vi "trmm - Triangle Matrix-Matrix Product.vi"   [LabVIEW 2020, in "NI_AALBLAS.lvlib"]
doc: "Calculates the product of a triangular matrix and another matrix."
uses:
  NI_AALBLAS.lvlib
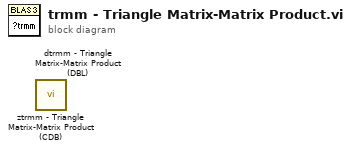
[diagram p0: block diagram]
diagram:
  n1 = call "ztrmm - Triangle Matrix-Matrix Product (CDB).vi"() -> ()  [unwired: 10 in, 2 out]
  n2 = call "dtrmm - Triangle Matrix-Matrix Product (DBL).vi"() -> ()  [unwired: 10 in, 2 out]
